vi "KM_appendline -- freq sweep.vi"(1 "freq":dbl[](array[numeric]), 2 "Vout(V)":cdb[](array[numeric]), 7 "Save frequency scan":path=path "C:/data/Ultrasound/birdcage/Hg1201/Test", 8 "read/write control":T1, 9 "name or relative path":string) -> ()   [LabVIEW 2016]
uses:
  KM_file -- read-write control.ctl
  file -- read-write control.ctl
  <vilib>/Utility/libraryn.llb/Check if File or Folder Exists.vi
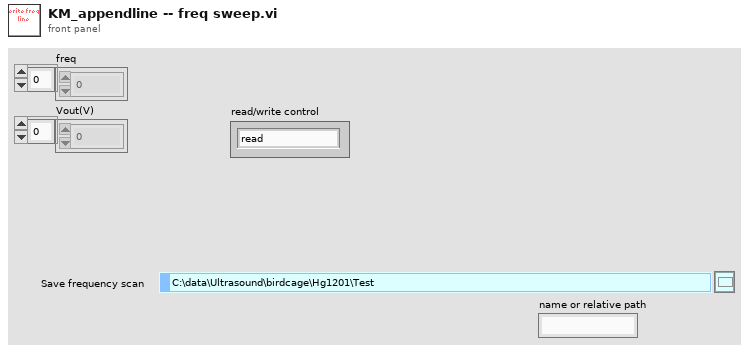
[diagram p1: front panel]
types:
  T1 = typedef "KM_file -- read-write control.ctl" = enum16{"read", "write all", "append one line"}
  T2 = typedef "file -- read-write control.ctl" = enum16{"read", "write all", "append one line"}
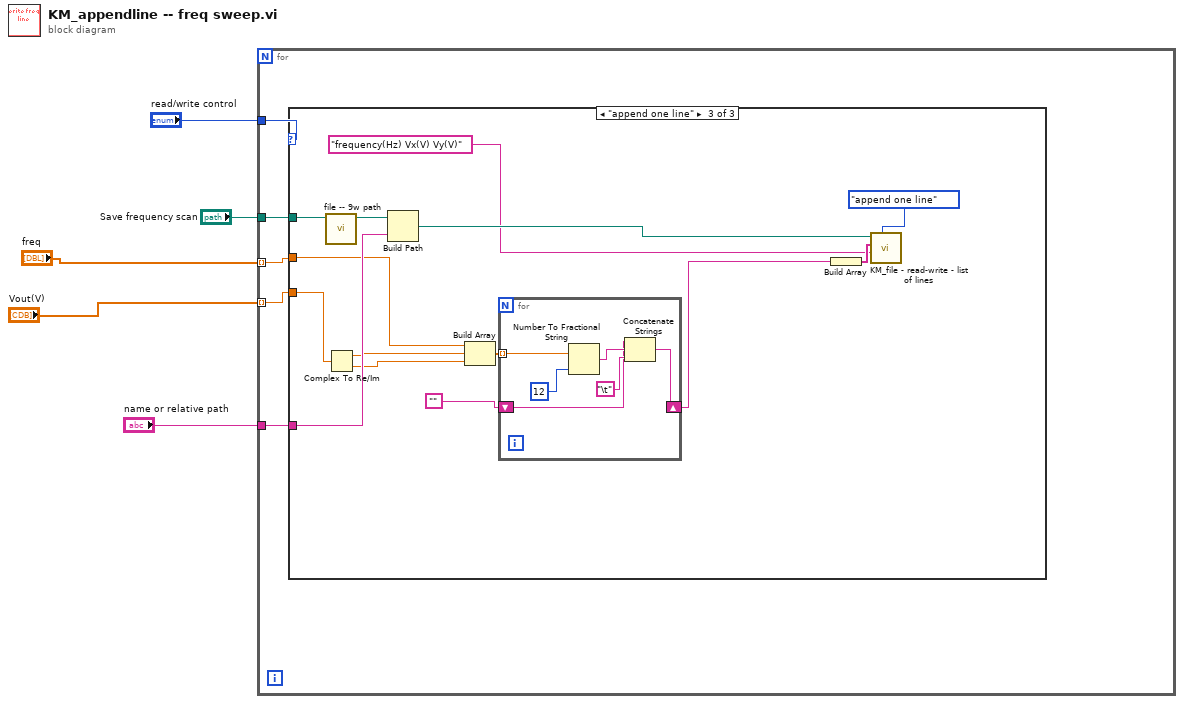
[diagram p0: block diagram]
diagram:
  n1 = for {
    tunnel: "read/write control" -> [w10]
    tunnel: "Save frequency scan" -> [w9]
    tunnel: "name or relative path" -> [w8]
    tunnel: "freq" -> [w7] mode=indexing
    tunnel: "Vout(V)" -> [w6] mode=indexing
    n2 = case shown="\"append one line\"" w10 {
      tunnel: w9 -> [_ _ w24]
      tunnel: w8 -> [_ _ w22]
      tunnel: w6 -> [_ _ w13]
      tunnel: w7 -> [_ _ w15]
      frame "read", Default {
      }
      frame "write all" {
      }
      frame "append one line" {
        n3 = call "file -- 9w path.vi"("sweep folder"=w24) -> ("9w path"=w23:path)  [unwired: 10 in]
        n4 = Complex To Re/Im(x + iy=w13) -> (x=w12:dbl, y=w11:dbl)
        n5 = Build Path(base path=w23, name or relative path=w22) -> (appended path=w17:path)
        n6 = Build Array(w15, w12, w11) -> (w21:dbl[])
        n7 = for {
          tunnel: w21 -> [w30] mode=indexing
          shift-right: [w26] -> w19
          shift-left: "" -> [w27]
          n8 = Number To Fractional String(number=w30, precision (6)=i16 12) -> (F-format string=w29:string)  [unwired: 2 in]
          n9 = Concatenate Strings(w27, w29, "\t" ("string")) -> (w26:string)
        }
        n10 = Build Array(w19) -> (w16:string[])
        n11 = call "KM_file - read-write - list of lines.vi"("read/write control"=file_--_read-write_control."append one line", "header"="frequency(Hz) Vx(V) Vy(V)", "list of lines IN"=w16, "file path"=w17) -> ()  [unwired: 6 in, 2 out]
      }
    }
  }
